vi "Agilent 34405 Read Single.vi"() -> ()   [LabVIEW 2018]
doc: "This example shows how to configure a measurement and take a single reading."
uses:
  <instrlib>/Agilent 34405/Agilent 34405.lvlib
panel:
  in  "Function (0: DC Volts)":i32(ring) items=["DC Volts", "AC Volts", "DC Current", "AC Current", "2-Wire Resistance", "Frequency", "Temperature", "Capacitance", "Continuity", "Diode", "4-Wire Resistance", "2nd DC Volts", "2nd AC Volts", "2nd DC Current", "2nd AC Current", "2nd Frequency"]
  in  "Manual Range (1)":dbl=1.0
  in  "Manual Resolution (5.5 Digits)":dbl(ring)=5.5 items=["3.5"=3.5, "4.5"=4.5, "5.5"=5.5]
  in  "Enable Auto Range (T:Enable)":bool=TRUE
  out "Measurement":dbl
  in  "VISA resource name":refnum<visa-resource-name>
  # "(c) 2009 - 2015 National Instruments Corporation.  ALL RIGHTS RESERVED."
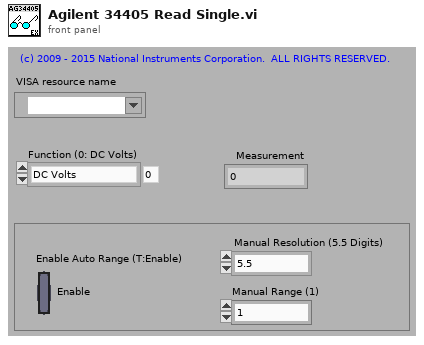
[diagram p1: front panel]
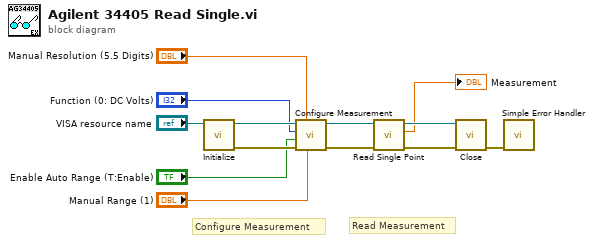
[diagram p0: block diagram]
diagram:
  # "Read Measurement"
  # "Configure Measurement"
  n1 = call <instrlib>:"Initialize.vi"("VISA resource name"="VISA resource name") -> ("error out"=w10:errorcluster, "VISA resource name out"=w11:refnum<visa-resource-name>)  [unwired: 3 in, 6 out]
  n2 = call <instrlib>:"Configure Measurement.vi"("Manual Range (1)"="Manual Range (1)", "Manual Resolution (5.5 Digits)"="Manual Resolution (5.5 Digits)", "error in (no error)"=w10, "Enable Auto Range (T:Enable)"="Enable Auto Range (T:Enable)", "Function (0: DC Volts)"="Function (0: DC Volts)", "VISA resource name"=w11) -> ("error out"=w6:errorcluster, "VISA resource name out"=w7:refnum<visa-resource-name>)  [unwired: 4 out]
  n3 = call <instrlib>:"Read Single Point.vi"("error in (no error)"=w6, "VISA resource name"=w7) -> ("error out"=w9:errorcluster, "Measurement"=→"Measurement":dbl, "VISA resource name out"=w8:refnum<visa-resource-name>)  [unwired: 7 out]
  n4 = call <instrlib>:"Close.vi"("error in (no error)"=w9, "VISA resource name"=w8) -> ("error out"=w13:errorcluster)  [unwired: 9 out]
  n5 = call <vilib>:"Simple Error Handler.vi"("error in (no error)"=w13) -> ()  [unwired: 1 in, 8 out]
